vi "Insert Into Wire.vi"(8 "error in (no error)":errorcluster, 9 "Wire Source Term":refnum<vi>, 10 "Output Term":refnum<vi>, 11 "Input Term":refnum<vi>) -> (0 "error out":errorcluster)   [LabVIEW 2014]
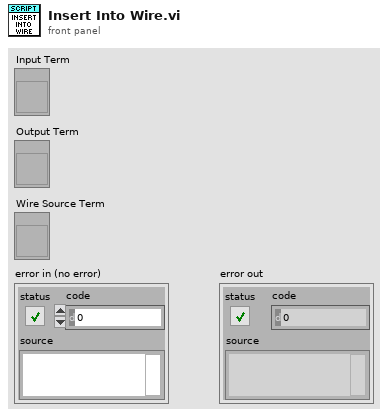
[diagram p1: front panel]
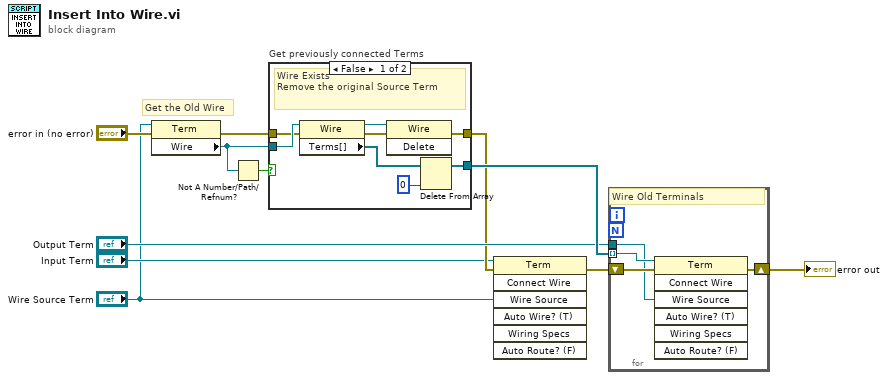
[diagram p0: block diagram]
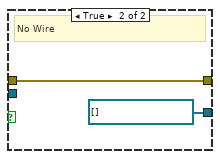
[diagram p2: hidden frame]
diagram:
  # "Get the Old Wire"
  n1 = property class="Term"(reference="Wire Source Term", error in="error in (no error)") -> (error out=w4:errorcluster, "Wire"=w3:refnum<vi>)  [unwired: 1 out]
  n2 = Not A Number/Path/Refnum?(number/path/refnum=w3) -> (NaN/Path/Refnum?=w2:bool)
  n3 = case "Get previously connected Terms" shown="False" w2 {
    tunnel: [w15 refnum<vi>[] [] ("Terms[]")] -> w10
    tunnel: [w14 w21] -> w8
    tunnel: w3 -> [w13 _]
    tunnel: w4 -> [w12 w21]
    frame False {
      # "Wire Exists\nRemove the original Source Term"
      n4 = property class="Wire"(reference=w13, error in=w12) -> (reference out=w19:refnum<vi>, error out=w18:errorcluster, "Terms[]"=w17:refnum<vi>[])
      n5 = invoke class="Wire" method="Delete"(reference=w19, error in=w18) -> (error out=w14:errorcluster)  [unwired: 1 in, 2 out]
      n6 = Delete From Array(array=w17, index=0) -> (array with subset deleted=w15:refnum<vi>[])  [unwired: 1 in, 1 out]
    }
    frame True {
      # "No Wire"
    }
  }
  n7 = invoke class="Term" method="Connect Wire"(reference="Input Term", error in=w8, "Wire Source"="Wire Source Term") -> (error out=w7:errorcluster)  [unwired: 4 in, 6 out]
  n8 = for {
    shift-right: [w25] -> w11
    shift-left: w7 -> [w24]
    tunnel: w10 -> [w23] mode=indexing
    tunnel: "Output Term" -> [w22]
    # "Wire Old Terminals"
    n9 = invoke class="Term" method="Connect Wire"(reference=w23, error in=w24, "Wire Source"=w22) -> (error out=w25:errorcluster)  [unwired: 4 in, 6 out]
  }
  "error out" <- w11
